vi "Is Flat Type.vi"(8 "error in (no error)":errorcluster, 11 "LVType in":refnum<class "LVType.lvclass">) -> (0 "error out":errorcluster, 2 "Flat Type?":bool=TRUE, 3 "LVType out":refnum<class "LVType.lvclass">)   [LabVIEW 2020, in "LVDataTypes.lvlib" / "LVType.lvclass"]
uses:
  <vilib>/AppBuilder/Engine/WebServiceDescription/LVDataTypes/LVType/LVType.lvclass
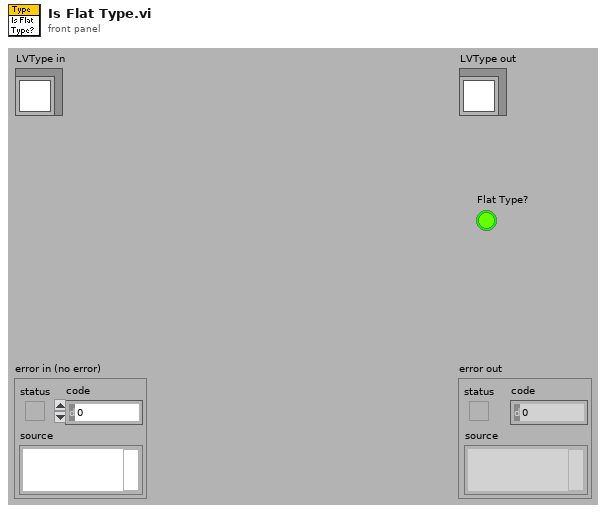
[diagram p1: front panel]
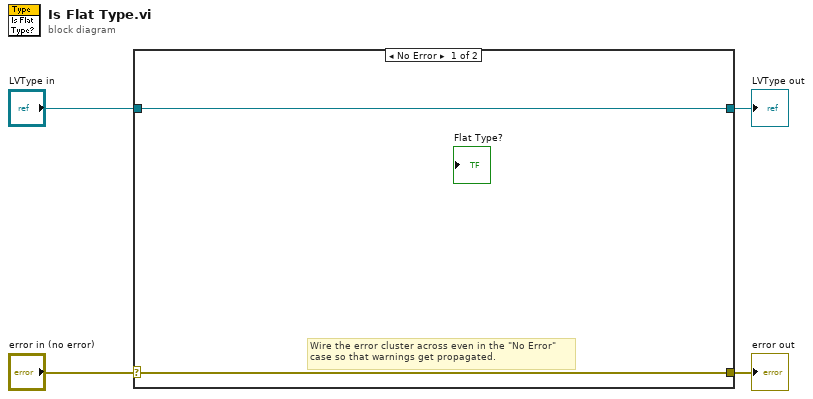
[diagram p0: block diagram]
diagram:
  n1 = case shown="No Error" "error in (no error)" {
    selector: "error in (no error)" -> [w5 w8]
    tunnel: [w5 w8] -> w3
    tunnel: [w6 w7] -> w1
    tunnel: "LVType in" -> [w6 w7]
    frame No Error {
      # "Wire the error cluster across even in the \"No Error\"\ncase so that warnings get propagated."
    }
    frame Error {
    }
  }
  "error out" <- w3
  "LVType out" <- w1
